vi "shutDownCamera.vi"(8 "error in (no error)":errorcluster, 10 "Log in":refnum<class "Log.lvclass">, 11 "AndorController in":refnum<class "AndorController.lvclass">) -> (0 "error out":errorcluster, 2 "Log out":refnum<class "Log.lvclass">, 3 "AndorController out":refnum<class "AndorController.lvclass">)   [LabVIEW 2009, in "Hardware.lvlib" / "Channels.lvlib" / "AndorController.lvclass"]
uses:
  AndorController.lvclass
  Tools/Log.lvclass
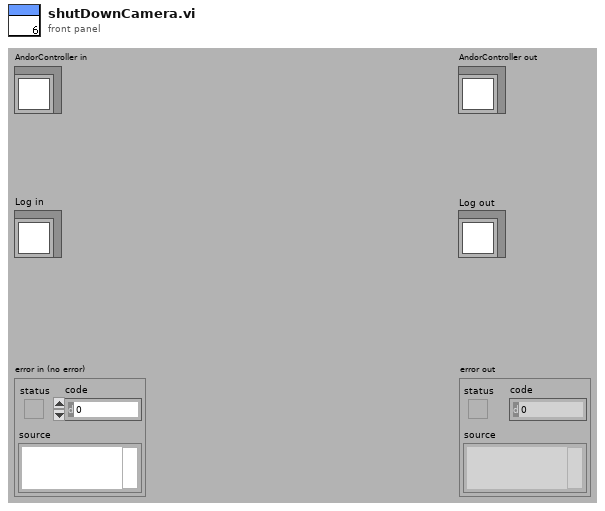
[diagram p1: front panel]
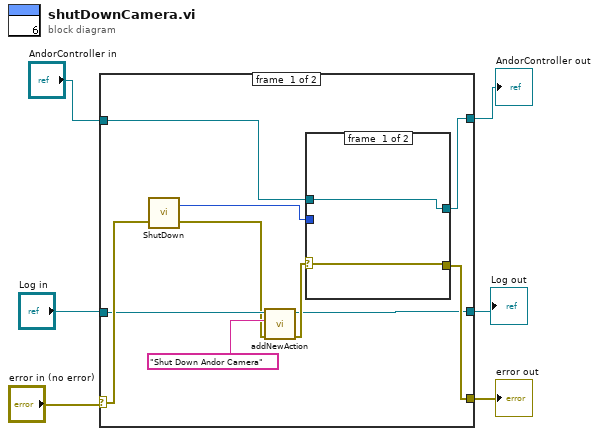
[diagram p0: block diagram]
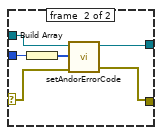
[diagram p2: hidden frame]
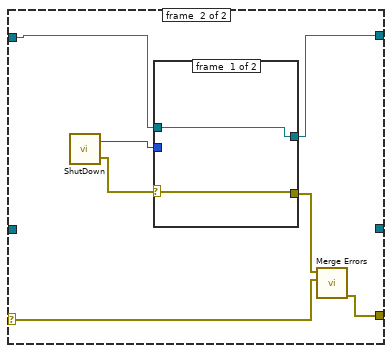
[diagram p3: hidden frame]
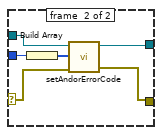
[diagram p4: hidden frame]
diagram:
  n1 = case shown="No Error" "error in (no error)" {
    selector: "error in (no error)" -> [w16 w26]
    tunnel: "AndorController in" -> [w14 w30]
    tunnel: [w13 w29] -> w4
    tunnel: [w12 w25] -> w3
    tunnel: "Log in" -> [w11 _]
    tunnel: [w7 _] -> w1
    frame #0 {
      n2 = call <userlib>:"ShutDown.vi"("error in (no error)"=w16) -> ("error out"=w9:errorcluster, "DLL error code"=w15:u32)  [unwired: 1 in]
      n3 = call-dynamic "addNewAction.vi"("error in (no error)"=w9, "newAction"="Shut Down Andor Camera", "Log in"=w11) -> ("error out"=w8:errorcluster, "Log out"=w7:refnum<class "Log.lvclass">)  [unwired: 7 in]
      n4 = case shown="Error" w8 {
        selector: w8 -> [w18 w23]
        tunnel: [w17 w24] -> w13
        tunnel: w15 -> [_ w21]
        tunnel: [w18 w22] -> w12
        tunnel: w14 -> [w17 w19]
        frame #0 {
        }
        frame #1 {
          n5 = Build Array(w21) -> (w20:u32[])
          n6 = call "setAndorErrorCode.vi"("error in (no error)"=w23, "Andor Error Codes"=w20, "AndorController.lvclass in"=w19) -> ("error out"=w22:errorcluster, "AndorController.lvclass out"=w24:refnum<class "AndorController.lvclass">)  [unwired: 7 in]
        }
      }
    }
    frame #1 {
      n7 = call <userlib>:"ShutDown.vi"() -> ("error out"=w28:errorcluster, "DLL error code"=w31:u32)  [unwired: 2 in]
      n8 = case shown="Error" w28 {
        selector: w28 -> [w33 w38]
        tunnel: [w32 w39] -> w29
        tunnel: w31 -> [_ w36]
        tunnel: [w33 w37] -> w27
        tunnel: w30 -> [w32 w34]
        frame #0 {
        }
        frame #1 {
          n9 = Build Array(w36) -> (w35:u32[])
          n10 = call "setAndorErrorCode.vi"("error in (no error)"=w38, "Andor Error Codes"=w35, "AndorController.lvclass in"=w34) -> ("error out"=w37:errorcluster, "AndorController.lvclass out"=w39:refnum<class "AndorController.lvclass">)  [unwired: 7 in]
        }
      }
      n11 = call <vilib>:"Merge Errors.vi"("error in 2 (no error)"=w26, "error in 1 (no error)"=w27) -> ("error out"=w25:errorcluster)  [unwired: 5 in]
    }
  }
  "error out" <- w3
  "AndorController out" <- w4
  "Log out" <- w1
